vi "UpdateACC.vi"(5 "Fall check ref":refnum<k24>, 7 "Strict refs box":T1, 8 "error in (no error)":errorcluster, 11 "BLE Message in":refnum<class "BLE Message.lvclass">) -> (0 "error out":errorcluster, 3 "BLE Message out":refnum<class "BLE Message.lvclass">)   [LabVIEW 2015, in "BLE Message.lvclass"]
uses:
  BLE Message.lvclass
  ctrls/RefsBox.ctl
  C:/Users/Bartek/Desktop/NORDIC/NORDIC LabVIEW GUI/DLLs/NordicDatabaseDLL.dll
  DLLs/NordicDatabaseDLL.dll
  BLE Message.lvclass/BLE Message.ctl
panel:
  out "size(s)":i32
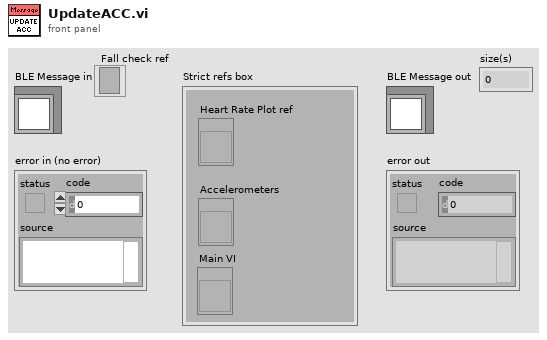
[diagram p1: front panel]
types:
  T1 = typedef "RefsBox.ctl" = cluster{"Heart Rate Plot ref":refnum<vi>, "Accelerometers":refnum<vi>, "Main VI":refnum<vi>}
  T2 = typedef "AccelerometerData.ctl" = cluster{"X":dbl, "Y":dbl, "Z":dbl}
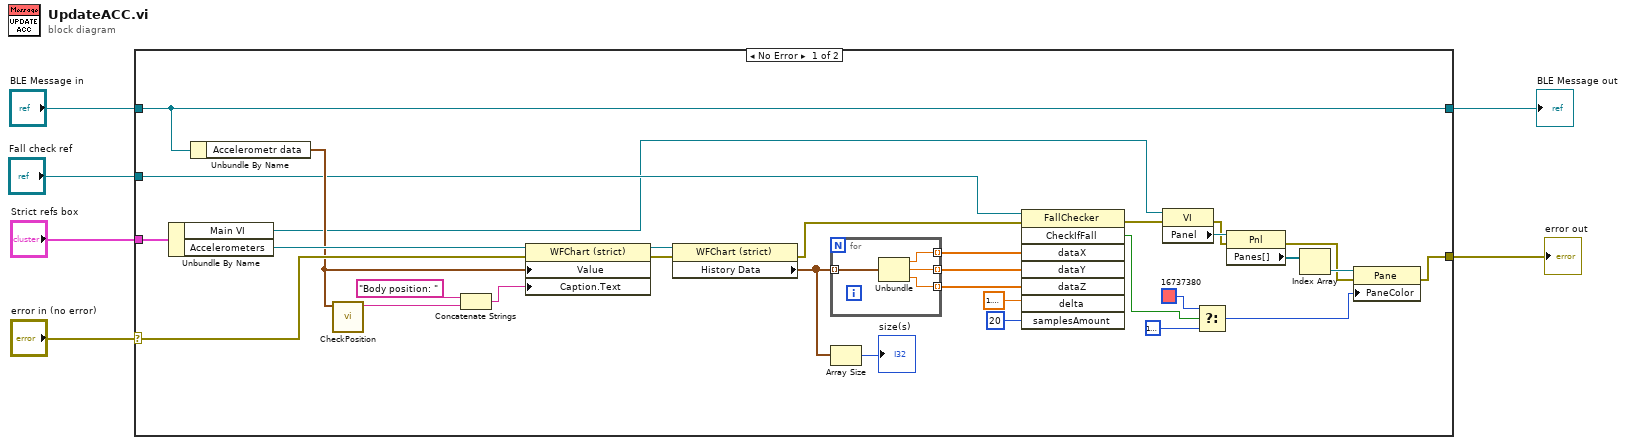
[diagram p0: block diagram]
diagram:
  n1 = case shown="No Error" "error in (no error)" {
    selector: "error in (no error)" -> [w34 w43]
    tunnel: [w16 w43] -> w5
    tunnel: [w35 w42] -> w3
    tunnel: "BLE Message in" -> [w35 w42]
    tunnel: "Strict refs box" -> [w37 _]
    tunnel: "Fall check ref" -> [w27 _]
    frame No Error {
      n2 = Unbundle By Name(w37) -> ("Main VI"=w22:refnum<vi>, "Accelerometers"=w36:refnum<vi>)
      n3 = Unbundle By Name(w35) -> ("Accelerometr data"=w30:T2)
      n4 = call "CheckPosition.vi"("Accelerometr data"=w30) -> ("State"=w33:string)  [unwired: 10 in]
      n5 = Concatenate Strings("Body position: " ("string"), w33) -> (w32:string)
      n6 = property class="WFChart (strict)"(reference=w36, error in=w34, "Value"=w30, "Caption.Text"=w32) -> (reference out=w28:refnum<vi>, error out=w29:errorcluster)
      n7 = property class="WFChart (strict)"(reference=w28, error in=w29) -> (error out=w26:errorcluster, "History Data"=w8:cluster{dbl, dbl, dbl}[])  [unwired: 1 out]
      n8 = for {
        tunnel: w8 -> [w41] mode=indexing
        tunnel: [w40] -> w25 mode=indexing
        tunnel: [w39] -> w24 mode=indexing
        tunnel: [w38] -> w23 mode=indexing
        n9 = Unbundle(w41) -> (w40:dbl, w39:dbl, w38:dbl)
      }
      n10 = Array Size(array=w8) -> (size(s)=→"size(s)":i32)
      n11 = invoke class="FallChecker" method="CheckIfFall"(reference=w27, error in=w26, "dataX"=w25, "dataY"=w24, "dataZ"=w23, "delta"=sgl 1.4, "samplesAmount"=20) -> (error out=w13:errorcluster, "CheckIfFall"=w14:bool)  [unwired: 1 in, 6 out]
      n12 = property class="VI"(reference=w22, error in=w13) -> (error out=w20:errorcluster, "Panel"=w21:refnum<vi>)  [unwired: 1 out]
      n13 = Select(t=u32 16737380, s=w14, f=u32 16777238) -> (s? t:f=w11:u32)
      n14 = property class="Pnl"(reference=w21, error in=w20) -> (error out=w17:errorcluster, "Panes[]"=w19:refnum<vi>[])  [unwired: 1 out]
      n15 = Index Array(array=w19) -> (element=w18:refnum<vi>)  [unwired: 1 in]
      n16 = property class="Pane"(reference=w18, error in=w17, "PaneColor"=w11) -> (error out=w16:errorcluster)  [unwired: 1 out]
    }
    frame Error {
    }
  }
  "error out" <- w5
  "BLE Message out" <- w3
